vi "Place piece.vi"(8 "error in (no error)":errorcluster, 9 "Piece":T1, 10 "Square":T4={"File"=enum."a", "Rank"=enum."4"}, 11 "Board in":refnum<class "Board.lvclass">) -> (0 "error out":errorcluster, 1 "Removed piece":T1, 2 "Square occupied?":bool, 3 "Board out":refnum<class "Board.lvclass">)   [LabVIEW 2015, in "Chesslib.lvlib" / "Board.lvclass"]
uses:
  Board.lvclass
  typedef/Piece.ctl
  typedef/Color.ctl
  typedef/Piece type.ctl
  typedef/Square.ctl
  typedef/File.ctl
  typedef/Rank.ctl
  Chesslib.lvlib
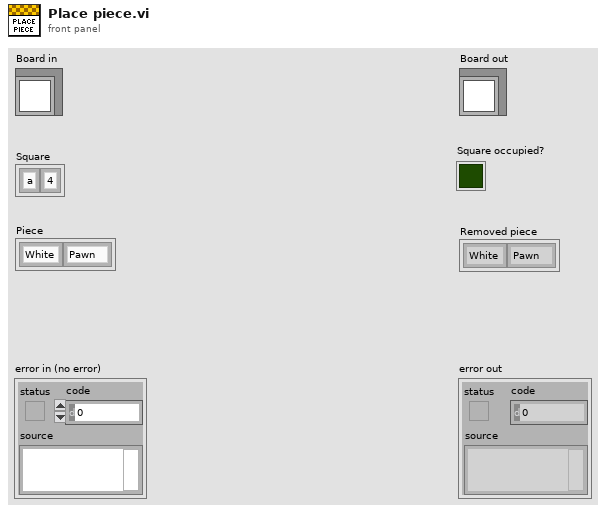
[diagram p1: front panel]
types:
  T1 = typedef "Chesslib.lvlib/Piece.ctl" = cluster{"Color":T2, "Type":T3}
  T2 = typedef "Chesslib.lvlib/Color.ctl" = enum16{"White", "Black"}
  T3 = typedef "Chesslib.lvlib/Piece type.ctl" = enum16{"Pawn", "Bishop", "Knight", "Rook", "Queen", "King"}
  T4 = typedef "Chesslib.lvlib/Square.ctl" = cluster{"File":T5, "Rank":T6}
  T5 = typedef "Chesslib.lvlib/File.ctl" = enum16{"a", "b", "c", "d", "e", "f", "g", "h"}
  T6 = typedef "Chesslib.lvlib/Rank.ctl" = enum16{"1", "2", "3", "4", "5", "6", "7", "8"}
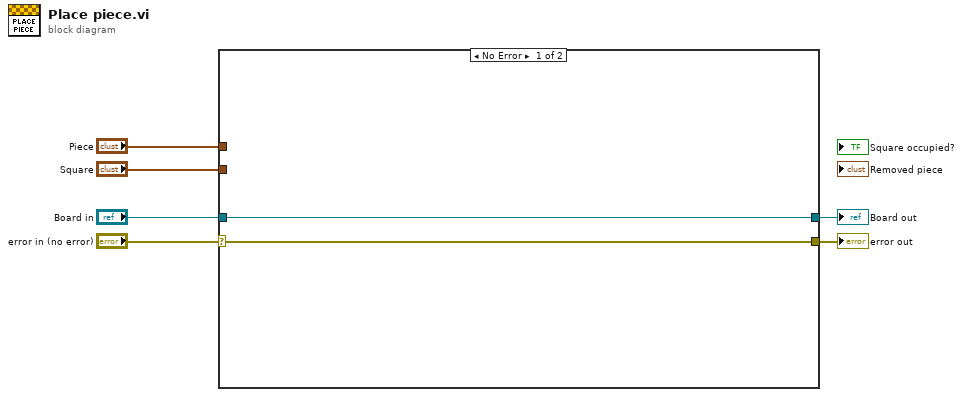
[diagram p0: block diagram]
diagram:
  n1 = case shown="No Error" "error in (no error)" {
    selector: "error in (no error)" -> [w8 w10]
    tunnel: [w8 w10] -> w5
    tunnel: [w7 w9] -> w3
    tunnel: "Board in" -> [w7 w9]
    tunnel: "Square" -> [_ _]
    tunnel: "Piece" -> [_ _]
    frame No Error {
    }
    frame Error {
    }
  }
  "error out" <- w5
  "Board out" <- w3
